vi "Configure Reference Oscillator.vi"(6 "External Frequency (10 MHz)":dbl=10000000.0, 7 "Internal BBG Frequency (10 MHz)":dbl=10000000.0, 8 "error in (no error)":errorcluster, 9 "External Bandwidth (25 Hz)":dbl=25.0, 10 "Internal Bandwidth (25 Hz)":dbl=25.0, 11 "VISA resource name":refnum<visa-resource-name>) -> (0 "error out":errorcluster, 3 "VISA resource name out":refnum<visa-resource-name>)   [LabVIEW 2014, in "Agilent PSG MXG Series.lvlib"]
doc: "Configures internal bandwidth, internal BBG frequency, external bandwidth and external frequency of the reference oscillator.\n\n<B>Notes:</B>\n(1) This VI is valid only in E8247C, E8257C, E8267C, E8257D, E8267D, N5161A, N5162A, N5181A, N5182A, N5183A, N5171B, N5172B, N5181B, N5182B."
uses:
  Agilent PSG MXG Series.lvlib
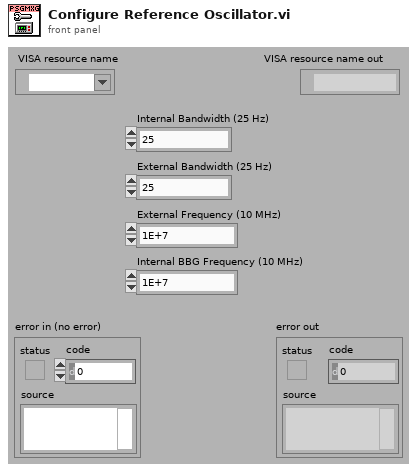
[diagram p1: front panel]
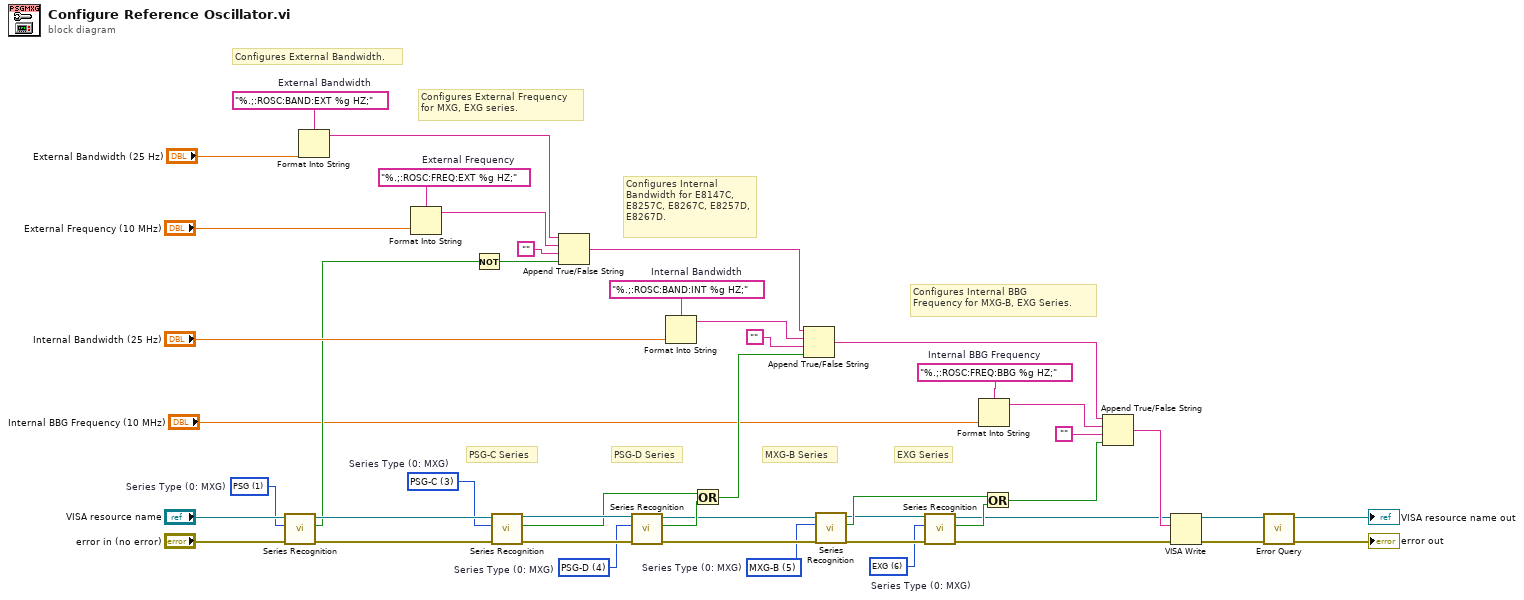
[diagram p0: block diagram]
diagram:
  w11 = u16 6 items=["MXG-A", "PSG", "PSG-A", "PSG-C", "PSG-D", "MXG-B", "EXG"]  # Series Type (0: MXG)
  w12 = u16 5 items=["MXG-A", "PSG", "PSG-A", "PSG-C", "PSG-D", "MXG-B", "EXG"]  # Series Type (0: MXG)
  w14 = "%.;:ROSC:FREQ:BBG %g HZ;"  # Internal BBG Frequency
  w21 = u16 4 items=["MXG-A", "PSG", "PSG-A", "PSG-C", "PSG-D", "MXG-B", "EXG"]  # Series Type (0: MXG)
  w25 = u16 3 items=["MXG-A", "PSG", "PSG-A", "PSG-C", "PSG-D", "MXG-B", "EXG"]  # Series Type (0: MXG)
  w31 = u16 1 items=["MXG-A", "PSG", "PSG-A", "PSG-C", "PSG-D", "MXG-B", "EXG"]  # Series Type (0: MXG)
  w41 = "%.;:ROSC:FREQ:EXT %g HZ;"  # External Frequency
  w39 = "%.;:ROSC:BAND:INT %g HZ;"  # Internal Bandwidth
  w45 = "%.;:ROSC:BAND:EXT %g HZ;"  # External Bandwidth
  # "EXG Series"
  # "MXG-B Series"
  # "Configures Internal BBG\nFrequency for MXG-B, EXG Series."
  # "PSG-D Series"
  # "PSG-C Series"
  # "Configures Internal\nBandwidth for E8147C,\nE8257C, E8267C, E8257D,\nE8267D."
  # "Configures External Frequency\nfor MXG, EXG series."
  # "Configures External Bandwidth."
  n1 = call "Series Recognition.vi"("error in (no error)"="error in (no error)", "Series Type (0: MXG)"=w31, "VISA resource name"="VISA resource name") -> ("error out"=w32:errorcluster, "Is Series Correct"=w26:bool, "VISA resource name out"=w34:refnum<visa-resource-name>)  [unwired: 1 in, 5 out]
  n2 = Format Into String(format string=w45, "External Bandwidth (25 Hz)") -> (resulting string=w30:string)  [unwired: 2 in, 1 out]
  n3 = Format Into String(format string=w41, "External Frequency (10 MHz)") -> (resulting string=w29:string)  [unwired: 2 in, 1 out]
  n4 = Not(x=w26) -> (.not. x?=w27:bool)
  n5 = call "Series Recognition.vi"("error in (no error)"=w32, "Series Type (0: MXG)"=w25, "VISA resource name"=w34) -> ("error out"=w23:errorcluster, "Is Series Correct"=w17:bool, "VISA resource name out"=w24:refnum<visa-resource-name>)  [unwired: 1 in, 5 out]
  n6 = Append True/False String(1:w27, 2:"", 3:w29, 4:w30) -> (0:w20:string)
  n7 = call "Series Recognition.vi"("error in (no error)"=w23, "Series Type (0: MXG)"=w21, "VISA resource name"=w24) -> ("error out"=w22:errorcluster, "Is Series Correct"=w18:bool, "VISA resource name out"=w3:refnum<visa-resource-name>)  [unwired: 1 in, 5 out]
  n8 = Format Into String(format string=w39, "Internal Bandwidth (25 Hz)") -> (resulting string=w19:string)  [unwired: 2 in, 1 out]
  n9 = Or(x=w17, y=w18) -> (x .or. y?=w16:bool)
  n10 = Append True/False String(1:w16, 2:"", 3:w19, 4:w20) -> (0:w8:string)
  n11 = call "Series Recognition.vi"("Series Type (0: MXG)"=w12, "VISA resource name"=w3) -> ("Is Series Correct"=w9:bool, "VISA resource name out"=w2:refnum<visa-resource-name>)  [unwired: 2 in, 6 out]
  n12 = call "Series Recognition.vi"("Series Type (0: MXG)"=w11, "VISA resource name"=w2) -> ("Is Series Correct"=w10:bool, "VISA resource name out"=w1:refnum<visa-resource-name>)  [unwired: 2 in, 6 out]
  n13 = Format Into String(format string=w14, "Internal BBG Frequency (10 MHz)") -> (resulting string=w7:string)  [unwired: 2 in, 1 out]
  n14 = Or(x=w9, y=w10) -> (x .or. y?=w5:bool)
  n15 = Append True/False String(1:w5, 2:"", 3:w7, 4:w8) -> (0:w4:string)
  n16 = VISA Write(VISA resource name=w1, write buffer=w4, error in (no error)=w22) -> (VISA resource name out=w44:refnum<visa-resource-name>, error out=w43:errorcluster)  [unwired: 1 out]
  n17 = call "Error Query.vi"("error in (no error)"=w43, "VISA resource name"=w44) -> ("error out"=→"error out":errorcluster, "VISA resource name out"=→"VISA resource name out":refnum<visa-resource-name>)  [unwired: 8 out]
